vi "Configure Edge Trigger.vi"(0 "RedPitaya connection in":refnum<k5>, 1 "Trigger Delay mode":enum16{"", "Samples", "Nanoseconds"}(ring), 2 "Delay (ns)":i32, 3 "Delay (# Samples)":i32 max=16348, 4 "Trigger Level (0 V)":dbl=20.1 min=-20.0 max=20.1, 5 "error in":errorcluster, 12 "timeout ms (2000)":i32=2000) -> (14 "RedPitaya connection out":refnum<k5>, 19 "error out":errorcluster)   [LabVIEW 2021, in "RedPitaya.lvlib"]
doc: "Configures edge trigger settings. An edge trigger occurs when the trigger signal passes through the voltage threshold that you specify with the <B>Trigger Level</B> control.\n\nTo set acquisition trigger delay first select units in which you want to set by input <b>Trigger Delay mode</b>."
uses:
  RedPitaya.lvlib
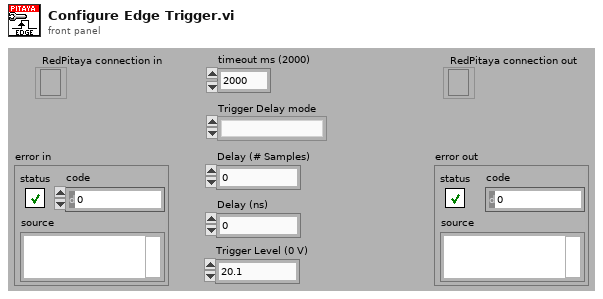
[diagram p1: front panel]
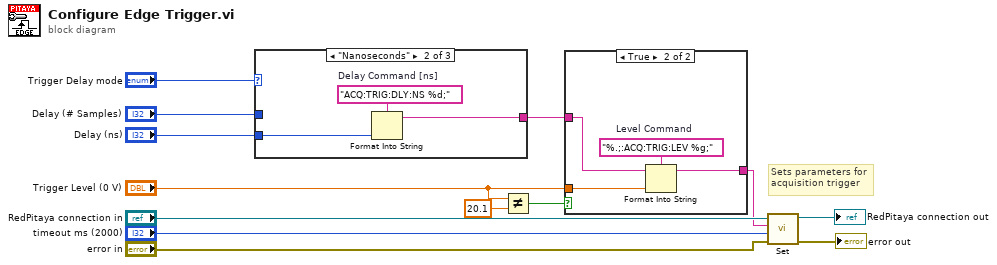
[diagram p0: block diagram]
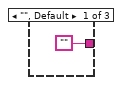
[diagram p3: hidden frame]
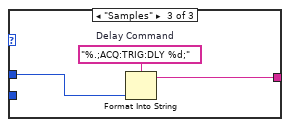
[diagram p4: hidden frame]
diagram:
  # "Sets parameters for\nacquisition trigger"
  n1 = case shown="\"Nanoseconds\"" "Trigger Delay mode" {
    tunnel: ["" w16 w19] -> w11
    tunnel: "Delay (ns)" -> [_ w15 _]
    tunnel: "Delay (# Samples)" -> [_ _ w18]
    frame "", Default {
    }
    frame "Nanoseconds" {
      w17 = "ACQ:TRIG:DLY:NS %d;"  # Delay Command [ns]
      n2 = Format Into String(format string=w17, w15) -> (resulting string=w16:string)  [unwired: 2 in, 1 out]
    }
    frame "Samples" {
      w20 = "%.;ACQ:TRIG:DLY %d;"  # Delay Command
      n3 = Format Into String(format string=w20, w18) -> (resulting string=w19:string)  [unwired: 2 in, 1 out]
    }
  }
  n4 = Not Equal?(x="Trigger Level (0 V)", y=20.1) -> (x != y?=w3:bool)
  n5 = case shown="True" w3 {
    tunnel: w11 -> [w21 w24]
    tunnel: [w21 w23] -> w6
    tunnel: "Trigger Level (0 V)" -> [_ w22]
    frame False {
    }
    frame True {
      w25 = "%.;:ACQ:TRIG:LEV %g;"  # Level Command
      n6 = Format Into String(format string=w25, initial string=w24, w22) -> (resulting string=w23:string)  [unwired: 1 in, 1 out]
    }
  }
  n7 = call "Set.vi"("error in"="error in", "timeout ms (2000)"="timeout ms (2000)", "SCPI Message"=w6, "RedPitaya connection in"="RedPitaya connection in") -> ("error out"=→"error out":errorcluster, "RedPitaya connection out"=→"RedPitaya connection out":refnum<k5>)  [unwired: 5 in, 1 out]
